vi "Gear Teleop.vi"(0 "Cluster":T1={"Axes Right"=[], " Axes Left"=[], " Axes Co-driver"=[0.0, 0.0, 0.0, 0.0, 0.0, 0.0], "Buttons Right"=[], "Buttons Left"=[], "Buttons Co-driver"=[FALSE, FALSE, FALSE, FALSE, FALSE, FALSE, FALSE, FALSE, FALSE, FALSE, FALSE], "POVs Right"=[], "POVs Left"=[], "POVs Co-driver"=[-1]}) -> ()   [LabVIEW 2016]
uses:
  Joystick vals.ctl
  <vilib>/Rock Robotics/WPI/Solenoid/WPI_SolenoidValue.ctl
  <vilib>/Rock Robotics/Network Tables/NT Write Boolean.vi
  <vilib>/Rock Robotics/WPI/Solenoid/WPI_SolenoidSetEnum.vi
  <vilib>/Rock Robotics/WPI/Solenoid/WPI_SolenoidGetEnum.vi
panel:
  in  "Outake":dbl=1.0
  in  "Intake":dbl=-1.0
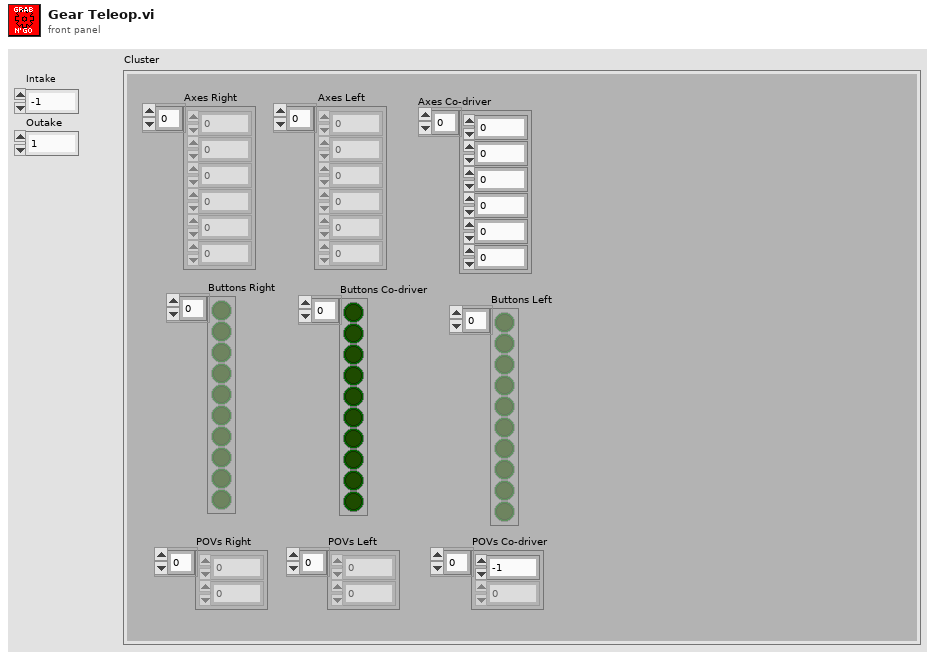
[diagram p1: front panel]
types:
  T1 = typedef "Joystick vals.ctl" = cluster{"Axes Right":dbl[], " Axes Left":dbl[], " Axes Co-driver":dbl[], "Buttons Right":bool[], "Buttons Left":bool[], "Buttons Co-driver":bool[], "POVs Right":i16[], "POVs Left":i16[], "POVs Co-driver":i16[]}
  T2 = typedef "WPI_MotorControlDeviceRef.ctl" = cluster{"DeviceStatus":errorcluster, "Type":T3, "PWM":cluster{"PWM Channel":T4, "DeadBand":T5}, "CAN":cluster{"Device Number":u8, "SetOutput VI Ref":variant, "GetOutput VI Ref":variant, "Enable VI Ref":variant, "Disable VI Ref":variant, "Data":variant}, "Invert":bool}
  T3 = typedef "WPI_MotorControlType.ctl" = enum16{"PWM", "CAN"}
  T4 = typedef "FPGA_DIOPWMChannel.ctl" = enum8{"PWM 0", "PWM 1", "PWM 2", "PWM 3", "PWM 4", "PWM 5", "PWM 6", "PWM 7", "PWM 8", "PWM 9", "PWM MXP 0", "PWM MXP 1", "PWM MXP 2", "PWM MXP 3", "PWM MXP 4", "PWM MXP 5", "PWM MXP 6", "PWM MXP 7", "PWM MXP 8", "PWM MXP 9", "Invalid"}
  T5 = typedef "WPI_PWMDeadband.ctl" = cluster{"Name":string, "maxPositivePwm":i32, "minPositivePwm":i32, "centerPwm":i32, "maxNegativePwm":i32, "minNegativePwm":i32, "angularRange":u16}
  T6 = typedef "WPI_SolenoidDevRef.ctl" = cluster{"DevStatus":errorcluster, "Pneumatics Control Module":u8, "Forward Solenoid Channel":T7, "Reverse Solenoid Channel":T7}
  T7 = typedef "WPI_SolenoidChannel.ctl" = enum8{"Solenoid 0", "Solenoid 1", "Solenoid 2", "Solenoid 3", "Solenoid 4", "Solenoid 5", "Solenoid 6", "Solenoid 7", "Invalid"}
  T8 = typedef "WPI_SolenoidValue.ctl" = enum16{"Off", "On", "Forward", "Reverse"}
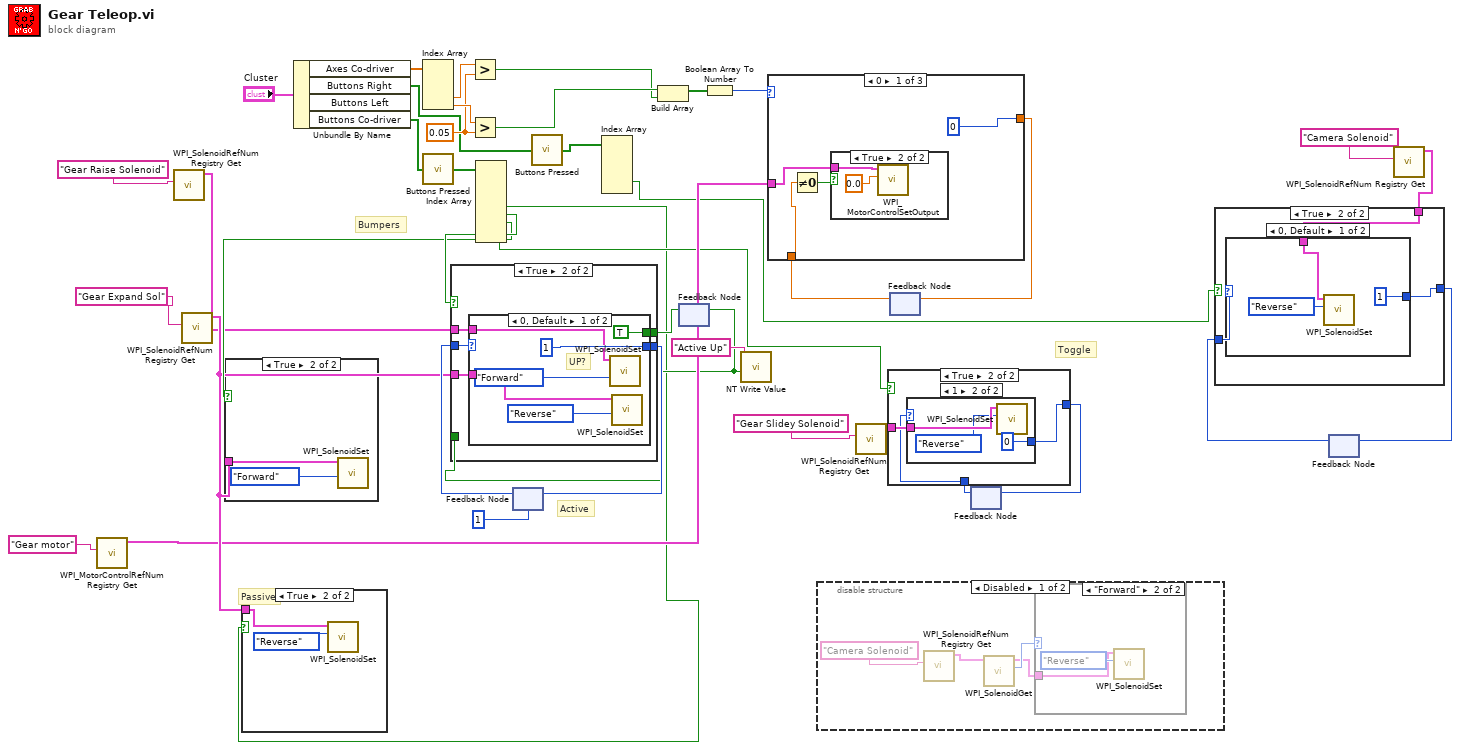
[diagram p0: block diagram]
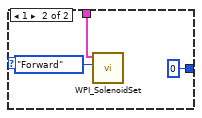
[diagram p3: hidden frame]
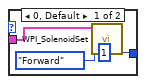
[diagram p5: hidden frame]
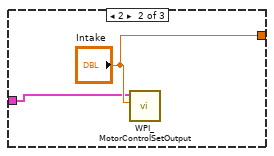
[diagram p11: hidden frame]
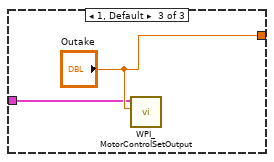
[diagram p12: hidden frame]
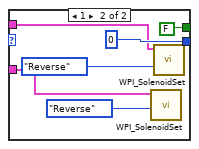
[diagram p14: hidden frame]
diagram:
  w33 = 0.05 ("y")
  # "Toggle"
  # "Bumpers"
  # "Passive"
  # "Active"
  n1 = call <vilib>:"WPI_MotorControlRefNum Registry Get.vi"("refnum name"="Gear motor") -> ("MotorControlDevRef"=w17:T2)  [unwired: 9 in, 1 out]
  n2 = call <vilib>:"WPI_SolenoidRefNum Registry Get.vi"("refnum name"="Gear Raise Solenoid") -> ("SolenoidDevRef"=w19:T6)  [unwired: 9 in, 1 out]
  n3 = call <vilib>:"WPI_SolenoidRefNum Registry Get.vi"("refnum name"="Gear Expand Sol") -> ("SolenoidDevRef"=w21:T6)  [unwired: 9 in, 1 out]
  n4 = Unbundle By Name("Cluster") -> ("Axes Co-driver"=w36:dbl[], "Buttons Right"=w4:bool[], "Buttons Co-driver"=w32:bool[])  [unwired: 1 out]
  n5 = Index Array(array=w36) -> (element #3=w35:dbl, element #4=w34:dbl)  [unwired: 4 in, 2 out]
  n6 = call "Buttons Pressed.vi"("Button Values"=w32) -> ("Button Presses"=w31:bool[])
  n7 = Greater?(x=w35, y=w33) -> (0:w28:bool)
  n8 = Greater?(x=w34, y=w33) -> (0:w29:bool)
  n9 = Index Array(array=w31) -> (element #4=w1:bool, element #5=w39:bool, element #6=w25:bool, element #8=w14:bool)  [unwired: 8 in, 4 out]
  n10 = case shown="True" w25 {
    tunnel: w21 -> [_ w41]
    frame False {
    }
    frame True {
      n11 = call-poly <vilib>:"WPI_SolenoidSet.vi"("Value"=WPI_SolenoidValue."Forward", "SolenoidDevRef"=w41) -> ()  [unwired: 8 in, 2 out]
    }
  }
  n12 = case shown="True" w1 {
    tunnel: w21 -> [_ w43]
    frame False {
    }
    frame True {
      n13 = call-poly <vilib>:"WPI_SolenoidSet.vi"("Value"=WPI_SolenoidValue."Reverse", "SolenoidDevRef"=w43) -> ()  [unwired: 8 in, 2 out]
    }
  }
  n14 = feedback #1(1) -> (w37:i32)
  n15 = call "Buttons Pressed.vi"("Button Values"=w4) -> ("Button Presses"=w5:bool[])
  n16 = Index Array(array=w5) -> (element #4=w3:bool)  [unwired: 5 in, 4 out]
  n17 = Build Array(w29, w28) -> (w30:bool[])
  n18 = feedback #2() -> (w2:bool)  [unwired: 1 in]
  n19 = case shown="True" w39 {
    tunnel: w37 -> [w46 w51]
    tunnel: [w46 w50] -> w26
    tunnel: w21 -> [_ w49]
    tunnel: w19 -> [_ w48]
    tunnel: [w45 w47] -> w15
    tunnel: w2 -> [w45 _]
    frame False {
    }
    frame True {
      n20 = case shown="0, Default" w51 {
        tunnel: [1 0] -> w50
        tunnel: w49 -> [w55 w61]
        tunnel: w48 -> [w53 w58]
        tunnel: [TRUE FALSE] -> w47
        frame 0, Default {
          # "UP?"
          n21 = call-poly <vilib>:"WPI_SolenoidSet.vi"("Value"=WPI_SolenoidValue."Forward", "SolenoidDevRef"=w53) -> ()  [unwired: 8 in, 2 out]
          n22 = call-poly <vilib>:"WPI_SolenoidSet.vi"("Value"=WPI_SolenoidValue."Reverse", "SolenoidDevRef"=w55) -> ()  [unwired: 8 in, 2 out]
        }
        frame 1 {
          n23 = call-poly <vilib>:"WPI_SolenoidSet.vi"("Value"=WPI_SolenoidValue."Reverse", "SolenoidDevRef"=w61) -> ()  [unwired: 8 in, 2 out]
          n24 = call-poly <vilib>:"WPI_SolenoidSet.vi"("Value"=WPI_SolenoidValue."Reverse", "SolenoidDevRef"=w58) -> ()  [unwired: 8 in, 2 out]
        }
      }
    }
  }
  n25 = feedback-in #1(w26) -> ()
  n26 = feedback-in #2(w15) -> ()
  n27 = Boolean Array To Number(Boolean array=w30) -> (number=w27:u32)
  n28 = call-poly <vilib>:"NT Write Value.vi"("Boolean"=w2, "Name"="Active Up") -> ()  [unwired: 9 in, 1 out]
  n29 = disable-structure shown="Disabled" {
    frame Disabled {
      n30 = call <vilib>:"WPI_SolenoidRefNum Registry Get.vi"("refnum name"="Camera Solenoid") -> ("SolenoidDevRef"=w66:T6)  [unwired: 9 in, 1 out]
      n31 = call-poly <vilib>:"WPI_SolenoidGet.vi"("SolenoidDevRef"=w66) -> ("Value"=w65:T8, "SolenoidDevRef"=w64:T6)  [unwired: 8 in, 1 out]
      n32 = case shown="\"Forward\"" w65 {
        tunnel: w64 -> [_ w68]
        frame "Reverse", Default {
        }
        frame "Forward" {
          n33 = call-poly <vilib>:"WPI_SolenoidSet.vi"("Value"=WPI_SolenoidValue."Reverse", "SolenoidDevRef"=w68) -> ()  [unwired: 8 in, 2 out]
        }
      }
    }
    frame Enabled {
    }
  }
  n34 = call <vilib>:"WPI_SolenoidRefNum Registry Get.vi"("refnum name"="Gear Slidey Solenoid") -> ("SolenoidDevRef"=w12:T6)  [unwired: 9 in, 1 out]
  n35 = feedback #3() -> (w23:dbl)  [unwired: 1 in]
  n36 = case shown="0" w27 {
    tunnel: [0 "Intake" "Outake"] -> w24
    tunnel: w23 -> [w71 _ _]
    tunnel: w17 -> [w70 w76 w78]
    frame 0 {
      n37 = Not Equal To 0?(x=w71) -> (x != 0?=w73:bool)
      n38 = case shown="True" w73 {
        tunnel: w70 -> [_ w74]
        frame False {
        }
        frame True {
          n39 = call <vilib>:"WPI_MotorControlSetOutput.vi"("Output"=0.0, "MotorControlDevRef"=w74) -> ()  [unwired: 7 in, 3 out]
        }
      }
    }
    frame 2 {
      n40 = call <vilib>:"WPI_MotorControlSetOutput.vi"("Output"="Intake", "MotorControlDevRef"=w76) -> ()  [unwired: 7 in, 3 out]
    }
    frame 1, Default {
      n41 = call <vilib>:"WPI_MotorControlSetOutput.vi"("Output"="Outake", "MotorControlDevRef"=w78) -> ()  [unwired: 7 in, 3 out]
    }
  }
  n42 = feedback-in #3(w24) -> ()
  n43 = feedback #4() -> (w10:i32)  [unwired: 1 in]
  n44 = case shown="True" w14 {
    tunnel: w12 -> [_ w83]
    tunnel: [w80 w81] -> w11
    tunnel: w10 -> [w80 w82]
    frame False {
    }
    frame True {
      n45 = case shown="1" w82 {
        tunnel: w83 -> [w85 w89]
        tunnel: [1 0] -> w81
        frame 0, Default {
          n46 = call-poly <vilib>:"WPI_SolenoidSet.vi"("Value"=WPI_SolenoidValue."Forward", "SolenoidDevRef"=w85) -> ()  [unwired: 8 in, 2 out]
        }
        frame 1 {
          n47 = call-poly <vilib>:"WPI_SolenoidSet.vi"("Value"=WPI_SolenoidValue."Reverse", "SolenoidDevRef"=w89) -> ()  [unwired: 8 in, 2 out]
        }
      }
    }
  }
  n48 = feedback-in #4(w11) -> ()
  n49 = feedback #5() -> (w6:i32)  [unwired: 1 in]
  n50 = call <vilib>:"WPI_SolenoidRefNum Registry Get.vi"("refnum name"="Camera Solenoid") -> ("SolenoidDevRef"=w8:T6)  [unwired: 9 in, 1 out]
  n51 = case shown="True" w3 {
    tunnel: w8 -> [_ w91]
    tunnel: [w90 w93] -> w7
    tunnel: w6 -> [w90 w92]
    frame False {
    }
    frame True {
      n52 = case shown="0, Default" w92 {
        tunnel: [1 0] -> w93
        tunnel: w91 -> [w94 w98]
        frame 0, Default {
          n53 = call-poly <vilib>:"WPI_SolenoidSet.vi"("Value"=WPI_SolenoidValue."Reverse", "SolenoidDevRef"=w94) -> ()  [unwired: 8 in, 2 out]
        }
        frame 1 {
          n54 = call-poly <vilib>:"WPI_SolenoidSet.vi"("Value"=WPI_SolenoidValue."Forward", "SolenoidDevRef"=w98) -> ()  [unwired: 8 in, 2 out]
        }
      }
    }
  }
  n55 = feedback-in #5(w7) -> ()
